vi "3D-PosAdd.vi"() -> ()   [LabVIEW 2011]
panel:
  in  "Exit":bool
  in  "Add Pos":bool
  in  "Pos Name":string
  in  "Y Current Postion":string
  in  "X Current Postion":string
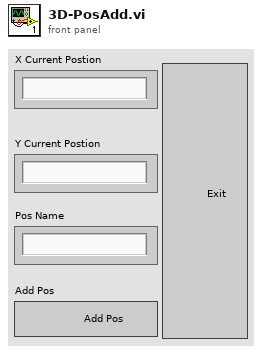
[diagram p1: front panel]
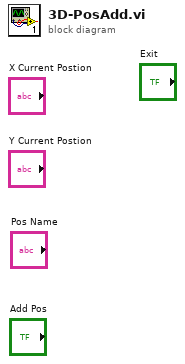
[diagram p0: block diagram]
diagram:
